vi "迭代器测试.vi"() -> ()   [LabVIEW 2011, in "迭代器.lvlib"]
panel:
  out "姓名":string
  out "Count":i32
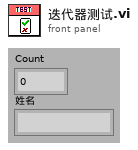
[diagram p1: front panel]
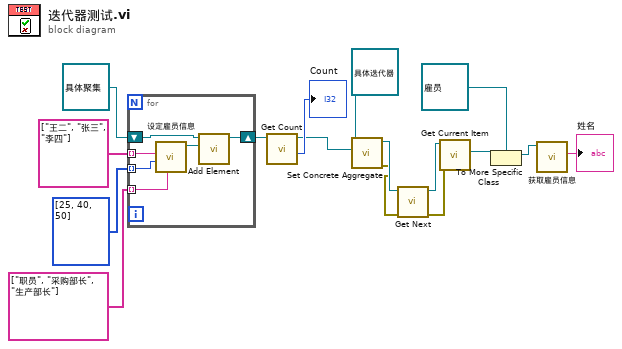
[diagram p0: block diagram]
diagram:
  n1 = for {
    tunnel: string[] ["王二", "张三", "李四"] -> [w22] mode=indexing
    tunnel: string[] ["职员", "采购部长", "生产部长"] -> [w21] mode=indexing
    tunnel: u8[] [25, 40, 50] -> [w20] mode=indexing
    shift-right: [w17] -> w11
    shift-left: refnum<class "具体聚集.lvclass"> refnum ("具体聚集 输入") -> [w19]
    n2 = call "设定雇员信息.vi"("职务"=w21, "年龄"=w20, "姓名"=w22) -> ("雇员 输出"=w18:refnum<class "雇员.lvclass">)  [unwired: 7 in, 1 out]
    n3 = call "Add Element.vi"("迭代器.lvlib:雇员.lvclass"=w18, "具体聚集 输入"=w19) -> ("具体聚集 输出"=w17:refnum<class "具体聚集.lvclass">)  [unwired: 8 in, 1 out]
  }
  n4 = call "Get Count.vi"("具体聚集 输入"=w11) -> ("Count"=→"Count":i32, "具体聚集 输出"=w10:refnum<class "具体聚集.lvclass">)  [unwired: 8 in, 1 out]
  n5 = call "Set Concrete Aggregate.vi"("迭代器.lvlib:具体聚集.lvclass"=w10, "具体迭代器 输入"=refnum<class "具体迭代器.lvclass"> refnum) -> ("error out"=w3:errorcluster, "具体迭代器 输出"=w4:refnum<class "具体迭代器.lvclass">)  [unwired: 8 in]
  n6 = call-dynamic "Get Next.vi"("error in (no error)"=w3, "Iterator(Abstract) 输入"=w4) -> ("error out"=w1:errorcluster, "Iterator(Abstract) 输出"=w2:refnum<class "具体迭代器.lvclass">)  [unwired: 7 in, 1 out]
  n7 = call-dynamic "Get Current Item.vi"("error in (no error)"=w1, "Iterator(Abstract) 输入"=w2) -> ("LabVIEW对象"=w9:refnum<class>)  [unwired: 7 in, 2 out]
  n8 = To More Specific Class(target class=refnum<class "雇员.lvclass"> refnum ("雇员 输入"), reference=w9) -> (specific class reference=w7:refnum<class "雇员.lvclass">)  [unwired: 1 in, 1 out]
  n9 = call-dynamic "获取雇员信息.vi"("雇员 输入"=w7) -> ("姓名"=→"姓名":string)  [unwired: 6 in, 4 out]
